vi "PH_IEEE1394Camera.get Cam.vi"(0 "i ref in":refnum<vi>, 5 "error in":errorcluster) -> (14 "i ref out":refnum<vi>, 16 "Cam found":bool, 18 "Cam Error out":errorcluster, 19 "error out":errorcluster)   [LabVIEW 2014, in "PH_IEEE1394Camera.lvlib"]
doc: "This VI is trying to connect to the cam which serial number is stored at the database. This number is expected to be the 64 Bit Hexadecimal number which one can get by the help of the MAX, or to be the serial number written on the cam. In the latter case this VI is restricted to 9 cams (cam0, cam1, ... cam8) only."
uses:
  PH_IEEE1394Camera.lvlib
  PH_Basics/PH_Common/PH_Common.lvlib
  PH_Basics/PH_Cam_BaseClass/PH_Cam_BaseClass.lvlib
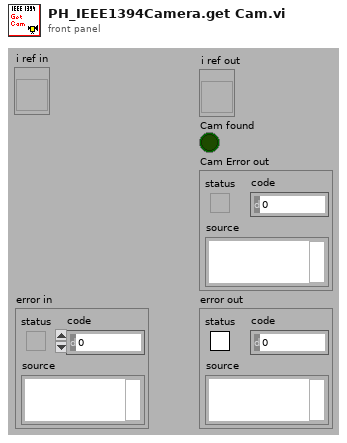
[diagram p1: front panel]
types:
  T1 = typedef "PH_Cam_BaseClass.lvlib/PH_Cam_BaseClass.i attribute.ctl" = cluster{"Gui Refs":T2, "Cam":cluster{"Source Notifier":refnum<notifier>, "Error":errorcluster, "Camera ID":string}, "Images":cluster{"Cam":T3, "Operation":T3, "PSDB":T3}, "Window Image":cluster{"Indicate Image":bool, "Window No.":i32, "Scale Facor":dbl, "Center Cross":bool, "Subtract Backgr":bool, "CoG":bool, "Color Palette":cluster{"Red":u8, "Green":u8, "Blue":u8}[], "Image On":bool}, "Default Prdc Int":i32, "Performance":cluster{"on":bool, "Timestamp Last Frame":i32}, "Histogram":cluster{"on":bool, "Mapping":bool}, "Save Image":cluster{"Save":bool, "File refnum":refnum<file>}, "Setting Service ID":i32, "Screen":cluster{"x-resolution":i16, "y-resolution":i16}, "On":bool, "Constructor finished":bool, "configured":bool}
  T2 = typedef "PH_Cam_BaseClass.lvlib/PH_Cam_BaseClass.GUI Refs.ctl" = cluster{"Frame Rate":refnum<vi>, "Get Frame Rate":refnum<vi>, "Show Image":refnum<vi>, "Get Histogram":refnum<vi>, "Mapping":refnum<vi>, "Histogram":refnum<vi>, "Center Cross":refnum<vi>, "Center of Gravity":refnum<vi>, "Scale Factor [%]":refnum<vi>, "Save Image":refnum<vi>, "Palette":refnum<vi>, "Subtract Background":refnum<vi>, "Cam Error":refnum<vi>, "On":refnum<vi>, "Cam List":refnum<vi>}
  T3 = typedef "IMAQ Image.ctl" = refnum<image>
  T4 = typedef "PH_IEEE1394Camera.lvlib/PH_IEEE1394Camera.i attribute.ctl" = cluster{"Gui Refs":cluster{"Brightness":refnum<vi>, "Shutter":refnum<vi>, "Gain":refnum<vi>, "Center of Gravity":refnum<vi>, "Supported Video Modes":refnum<vi>, "Trigger Polarity":refnum<vi>, "Trigger Mode":refnum<vi>, "Trigger Timeout":refnum<vi>, "Bit Depth":refnum<vi>, "Video Mode":refnum<vi>, "Top":refnum<vi>, "Bottom":refnum<vi>, "Left":refnum<vi>, "Right":refnum<vi>, "Set ROI to Maximum":refnum<vi>, "Camera Details":refnum<vi>, "Current Cam Attributes":refnum<vi>, "Attribute to set":refnum<vi>, "Num Value":refnum<vi>, "String Value":refnum<vi>, "Bool Value":refnum<vi>, "Set Cam Attribute":refnum<vi>}, "Cam":cluster{"IMAQ1394 Session":T5, "Camera Details":T6}, "Current Attributes":T7[], "Supported Video Modes ":cluster{"Video Mode":u32, "Video Mode Name":string}[], "Wanted Attributes":cluster{"Name":string, "Num Value":dbl, "String Value":string, "Boolean Value":bool}[], "Cam Attributes":T9}
  T5 = typedef "IMAQdx.ctl" = refnum<k21>
  T6 = typedef "PH_IEEE1394Camera.lvlib/PH_IEEE1394Camera.Cam Details.ctl" = cluster{"Model":string, "Serial Number":dbl, "Cam name (Machinery)":string, "Bus Type":string}
  T7 = typedef "PH_IEEE1394Camera.lvlib/PH_IEEE1394Camera.Cam Attribute.ctl" = cluster{"Information":cluster{"Type":T8, "Readable":bool, "Writable":bool, "Name":string}, "Num Value":dbl, "String Value":string, "Maximum":dbl, "Minimum":dbl, "Units":string, "Description":string, "EnumStrings[]":string[], "EnumValues[]":u32[], "Boolean Value":bool}
  T8 = typedef "NI_Vision_Acquisition_Software.lvlib/IMAQdx Attribute Type.ctl" = enum32{"U32", "I64", "DBL", "String", "Enum", "Bool", "Command"}
  T9 = typedef "PH_IEEE1394Camera.lvlib/PH_IEEE1394Camera.Relevant Cam Attributes.ctl" = cluster{"Video Mode":cluster{"Name":string, "Index":i32}, "Brightness":cluster{"Name":string, "Index":i32}, "Gain":cluster{"Name":string, "Index":i32}, "Shutter":cluster{"Name":string, "Index":i32}, "Trigger Pol":cluster{"Name":string, "Index":i32}, "Trigger Mode":cluster{"Name":string, "Index":i32}, "Timeout":cluster{"Name":string, "Index":i32}, "Bit Depth":cluster{"Name":string, "Index":i32}, "Pixel Bits":cluster{"Name":string, "Index":i32}, "Pixel Bytes":cluster{"Name":string, "Index":i32}, "Left":cluster{"Name":string, "Index":i32}, "Right":cluster{"Name":string, "Index":i32}, "Top":cluster{"Name":string, "Index":i32}, "Bottom":cluster{"Name":string, "Index":i32}}
  T10 = enum8{"Enabled", "Disabled", "Disabled and Grayed Out"}
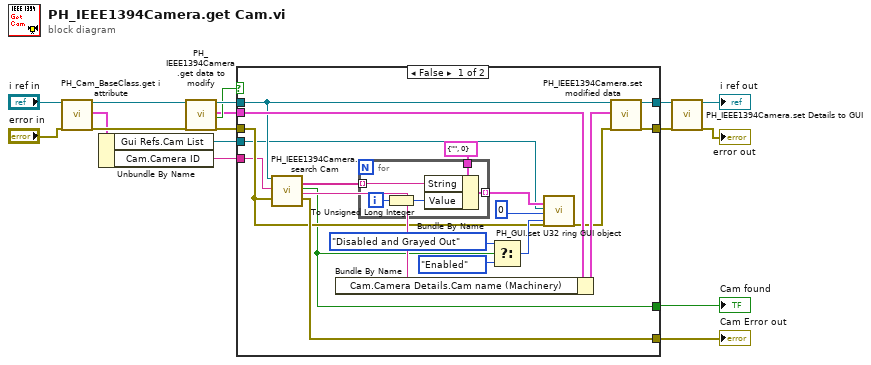
[diagram p0: block diagram]
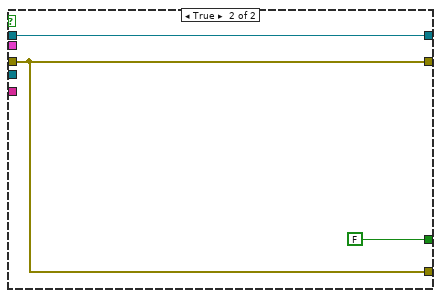
[diagram p2: hidden frame]
diagram:
  n1 = call "PH_Cam_BaseClass.get i attribute.vi"("i ref in"="i ref in", "error in (no error)"="error in") -> ("i ref out"=w8:refnum<vi>, "i attribute"=w7:T1, "error out"=w10:errorcluster)  [unwired: 15 in]
  n2 = Unbundle By Name(w7) -> ("Gui Refs.Cam List"=w5:refnum<vi>, "Cam.Camera ID"=w6:string)
  n3 = call "PH_IEEE1394Camera.get data to modify.vi"("i ref in"=w8, "error in (no error)"=w10) -> ("i ref out"=w16:refnum<vi>, "i attribute"=w14:T4, "timed out"=w15:bool, "error out"=w17:errorcluster)  [unwired: 14 in]
  n4 = case shown="False" w15 {
    tunnel: w17 -> [w22 w43]
    tunnel: w16 -> [w20 w44]
    tunnel: [w36 w44] -> w3
    tunnel: [w35 w43] -> w1
    tunnel: w14 -> [w33 _]
    tunnel: [w23 w43] -> w13
    tunnel: [w21 FALSE ("Cam found")] -> w12
    tunnel: w6 -> [w19 _]
    tunnel: w5 -> [w18 _]
    frame False {
      n5 = call "PH_IEEE1394Camera.search Cam.vi"("i ref in"=w20, "Cam ID (Serial Number)"=w19, "Cam Error in"=w22) -> ("Available Cams"=w25:string[], "Cam found"=w21:bool, "Cam.Name (machinery)"=w24:string, "Cam Error out"=w23:errorcluster)  [unwired: 13 in]
      n6 = Bundle By Name(cluster=w33, "Cam.Camera Details.Cam name (Machinery)"=w24) -> (w34:T4)
      n7 = for {
        tunnel: cluster{"String":string, "Value":u32} {"String"="", "Value"=0} -> [w41]
        tunnel: [w40] -> w32 mode=indexing
        tunnel: w25 -> [w37] mode=indexing
        i -> [w39]
        n8 = To Unsigned Long Integer(number=w39) -> (unsigned 32bit integer=w38:u32)
        n9 = Bundle By Name(cluster=w41, "String"=w37, "Value"=w38) -> (w40:cluster{"String":string, "Value":u32})
      }
      n10 = Select(t=T10."Disabled and Grayed Out" ("Disabled"), s=w21, f=T10."Enabled" ("Disabled")) -> (s? t:f=w27:T10)
      n11 = call "PH_GUI.set U32 ring GUI object.vi"("Strings And Values [Empty]"=w32, "Ring Ref"=w18, "Value"=u32 0, "error in (no error)"=w22, "Disabled (Enabled)"=w27) -> ("error out"=w26:errorcluster)  [unwired: 14 in]
      n12 = call "PH_IEEE1394Camera.set modified data.vi"("i ref in"=w20, "i attribute"=w34, "error in (no error)"=w26) -> ("i ref out"=w36:refnum<vi>, "error out"=w35:errorcluster)  [unwired: 15 in]
    }
    frame True {
    }
  }
  "Cam found" <- w12
  "Cam Error out" <- w13
  n13 = call "PH_IEEE1394Camera.set Details to GUI.vi"("VI in"=w3, "error in (no error)"=w1) -> ("VI out"=→"i ref out":refnum<vi>, "error out"=→"error out":errorcluster)  [unwired: 16 in]
